vi "LEBITplc.contents.vi"   [LabVIEW 2014, in "LEBITplc.lvlib"]
uses:
  LEBITplc.lvlib
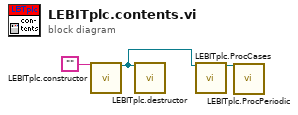
[diagram p0: block diagram]
diagram:
  n1 = call "LEBITplc.constructor.vi"("name"="") -> ("i ref out"=w2:refnum<vi>)  [unwired: 16 in, 2 out]
  n2 = call "LEBITplc.destructor.vi"("i ref in"=w2) -> ()  [unwired: 18 in, 1 out]
  n3 = call "LEBITplc.ProcCases.vi"("i ref in"=w2) -> ("i ref out"=w1:refnum<vi>)  [unwired: 16 in, 2 out]
  n4 = call "LEBITplc.ProcPeriodic.vi"("i ref in"=w1) -> ()  [unwired: 16 in, 3 out]
